vi "G#Object_Deserialize.vi"(0 "reference in":refnum<class "G#Interface.lvclass">, 1 "as xml (F)":bool, 2 "serialized object":string, 3 "class attributes (F)":bool, 4 "object id":u32[](array[numeric]), 5 "error in (no error)":errorcluster, 7 "include aggregates (T)":bool=TRUE) -> (14 "reference out":refnum<class "G#Interface.lvclass">, 18 "object id out":u32[](array[numeric]), 19 "error out":errorcluster)   [LabVIEW 2017, in "G#Interface.lvclass"]
doc: "Deserialize an object from a binary or XML string. XML implementation is a bit more robust since it could handle if serialization data doesn't exact match (if attributes has been added or removed)."
uses:
  <vilib>/addons/_AddQ/G#Interface/G#Interface.lvclass
  <vilib>/addons/_AddQ/G#Interface/G#Interface.lvclass/G#Interface.ctl
  <vilib>/addons/_AddQ/G#Object/G#Object.lvclass
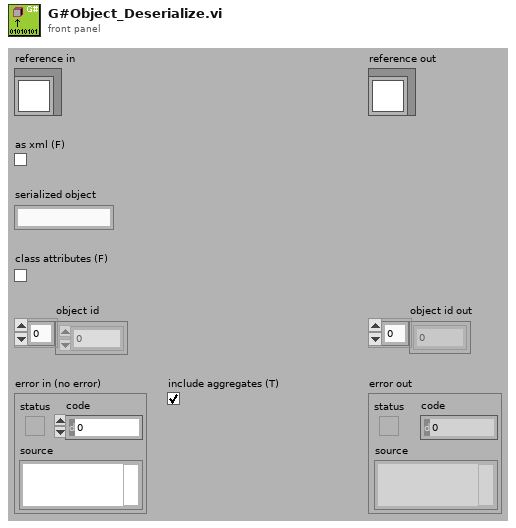
[diagram p1: front panel]
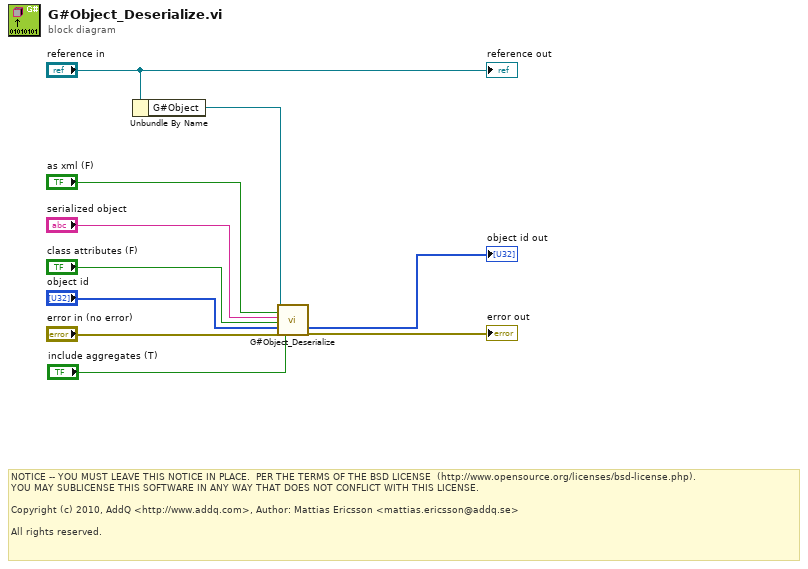
[diagram p0: block diagram]
diagram:
  # "NOTICE -- YOU MUST LEAVE THIS NOTICE IN PLACE.  PER THE TERMS OF THE BSD LICENSE  (http://www.opensource.org/licenses/bsd-license.php).\nYOU MAY SUBLICENSE THIS SOFTWARE IN ANY WAY THAT DOES NOT CONFLICT WITH THIS LICENSE.\n\nCopyright (c) 2010, AddQ <http://www.addq.com>, Author: Mattias Ericsson <mattias.ericsson@addq.se>\n\nAll rights reserved."
  n1 = Unbundle By Name("reference in") -> ("G#Object"=w6:refnum<class "G#Object.lvclass">)
  n2 = call-dynamic "G#Object_Deserialize.vi"("reference in"=w6, "as xml (F)"="as xml (F)", "serialized object"="serialized object", "class attributes (F)"="class attributes (F)", "object id"="object id", "error in (no error)"="error in (no error)", "include aggregates (T)"="include aggregates (T)") -> ("object id out"=→"object id out":u32[], "error out"=→"error out":errorcluster)  [unwired: 10 in, 1 out]
  "reference out" <- "reference in"
